vi "ClusterToDescriptiveStringGeneric.vi"(8 "error in":errorcluster, 11 "Cluster In":refnum<vi>) -> (0 "error out":errorcluster, 3 "String":string)   [LabVIEW 2023]
doc: "This VI turns a cluster (from reference) into a human/machine readable string."
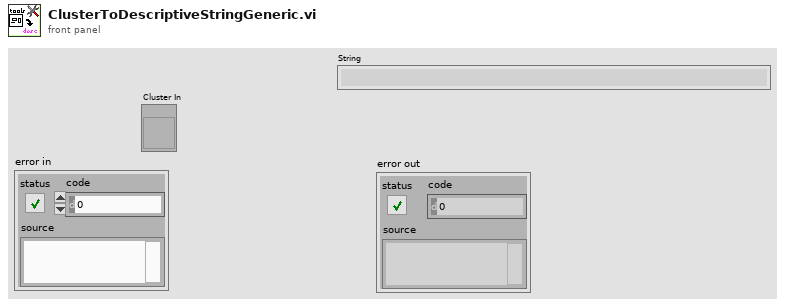
[diagram p1: front panel]
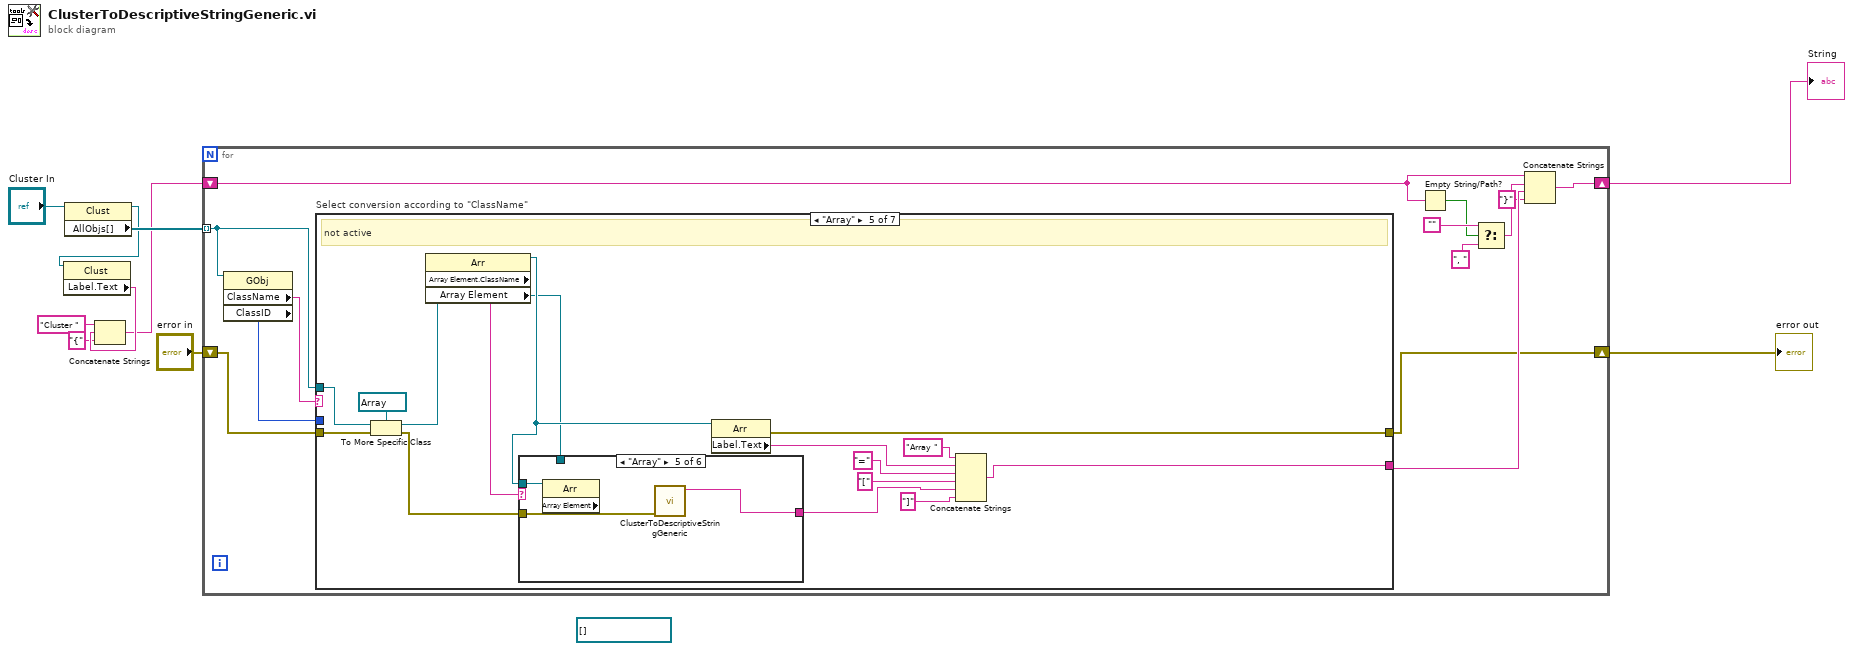
[diagram p0: block diagram]
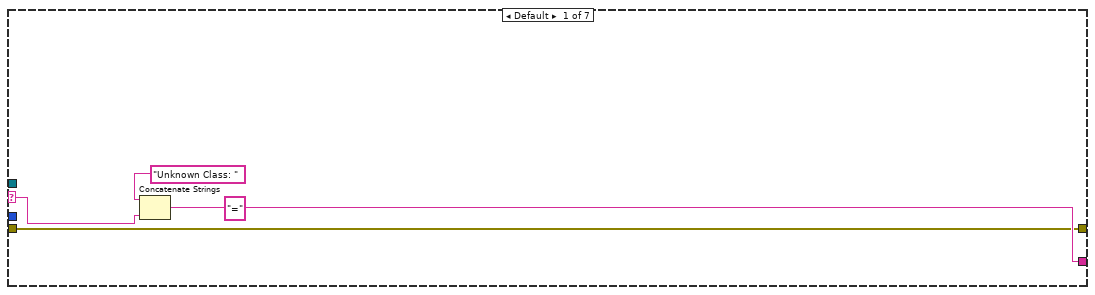
[diagram p2: hidden frame]
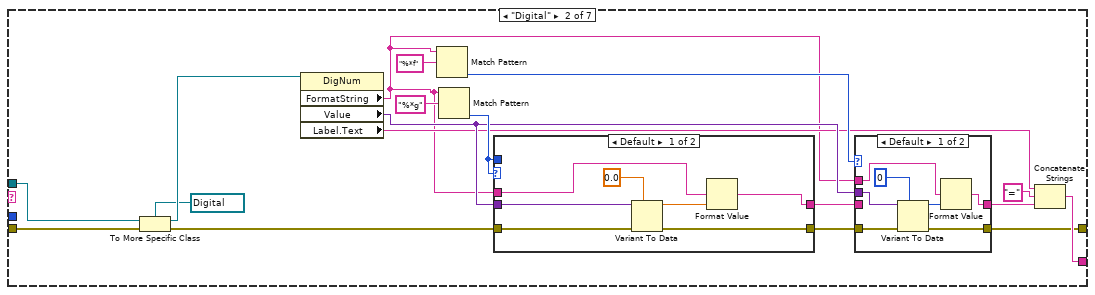
[diagram p3: hidden frame]
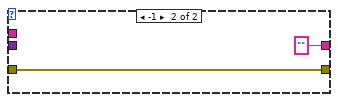
[diagram p5: hidden frame]
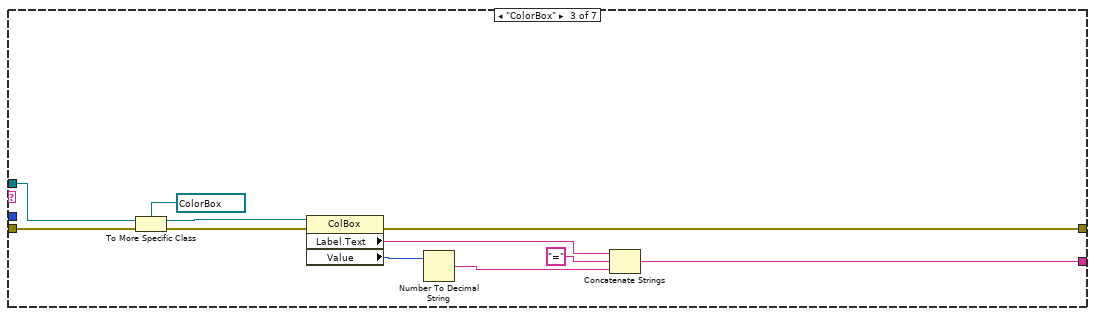
[diagram p6: hidden frame]
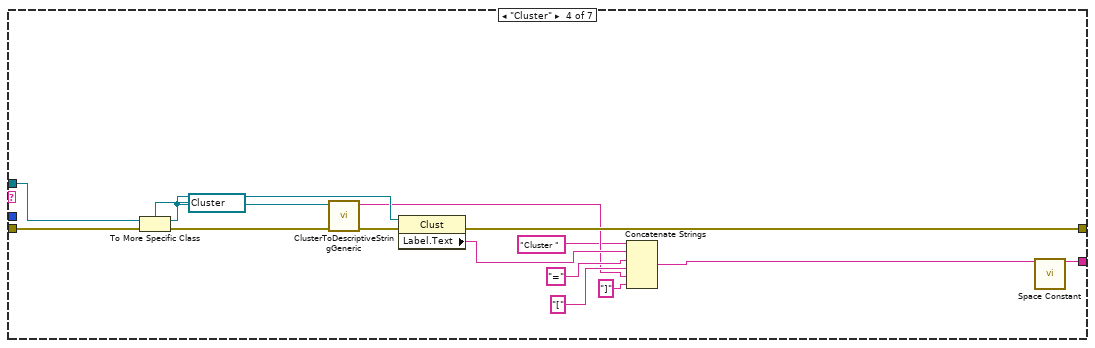
[diagram p7: hidden frame]
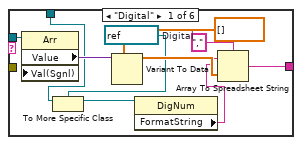
[diagram p8: hidden frame]
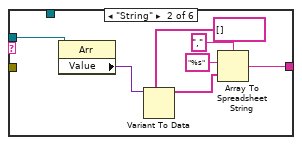
[diagram p9: hidden frame]
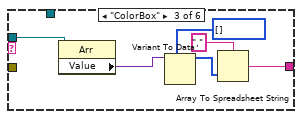
[diagram p10: hidden frame]
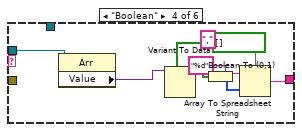
[diagram p11: hidden frame]
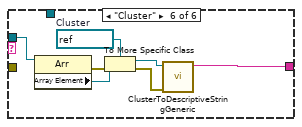
[diagram p12: hidden frame]
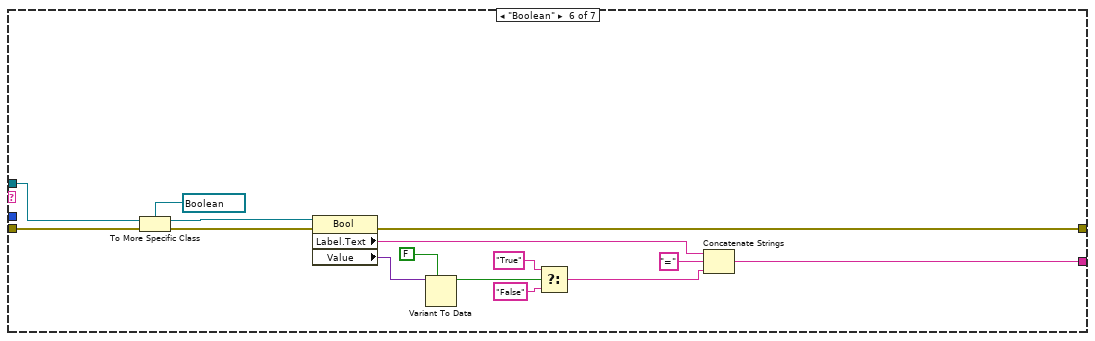
[diagram p13: hidden frame]
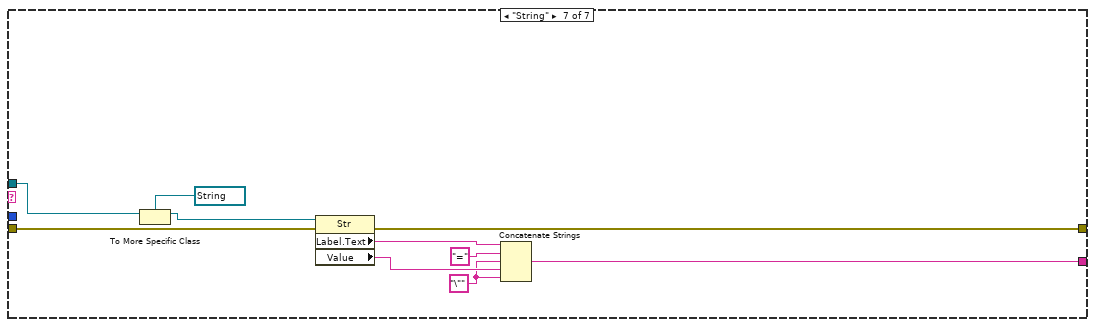
[diagram p14: hidden frame]
diagram:
  (unwired) refnum<vi>[] []
  n1 = property on="Property Node" class="Clust"(reference="Cluster In") -> (reference out=w5:refnum<vi>, "AllObjs[]"=w7:refnum<vi>[])  [unwired: 1 in, 1 out]
  n2 = property on="Property Node" class="Clust"(reference=w5) -> ("Label.Text"=w3:string)  [unwired: 1 in, 2 out]
  n3 = Concatenate Strings("Cluster " ("string"), w3, "{" ("string")) -> (w1:string)
  n4 = for {
    tunnel: w7 -> [w22] mode=indexing
    shift-right: [w23] -> w10
    shift-left: w1 -> [w13]
    shift-right: [w16] -> w8
    shift-left: "error in" -> [w15]
    n5 = property on="Property Node" class="GObj"(reference=w22) -> ("ClassName"=w20:string, "ClassID"=w21:u32)  [unwired: 1 in, 2 out]
    n6 = case "Select conversion according to \"ClassName\"" shown="\"Array\"" w20 {
      selector: w20 -> [w26 _ _ _ _ _ _]
      tunnel: [w25 w36 w71 w87 w103 w158 w169] -> w19
      tunnel: w22 -> [_ w46 w75 w89 w105 w161 w171]
      tunnel: w21 -> [_ _ _ _ _ _ _]
      tunnel: [w24 w30 w67 w84 w101 w149 w163] -> w16
      tunnel: w15 -> [w24 w33 w65 w83 w100 w147 w162]
      frame Default {
        n7 = Concatenate Strings("Unknown Class: ", "=", w26) -> (w25:string)
      }
      frame "Digital" {
        n8 = To More Specific Class(target class=refnum<vi> refnum ("567"), reference=w46, error in=w33) -> (specific class reference=w45:refnum<vi>, error out=w32:errorcluster)
        n9 = property on="Property Node" class="DigNum"(reference=w45) -> ("FormatString"=w35:string, "Value"=w42:variant, "Label.Text"=w38:string)  [unwired: 1 in, 2 out]
        n10 = Match Pattern(string=w35, regular expression="%*f") -> (offset past match=w39:i32)  [unwired: 1 in, 3 out]
        n11 = Match Pattern(string=w35, regular expression="%*g") -> (offset past match=w44:i32)  [unwired: 1 in, 3 out]
        n12 = case shown="Default" w44 {
          tunnel: w44 -> [_ _]
          tunnel: w42 -> [w62 _]
          tunnel: [w60 "" ("output string")] -> w43
          tunnel: w35 -> [w59 _]
          tunnel: w32 -> [w58 w63]
          tunnel: [w57 w63] -> w31
          frame Default {
            n13 = Variant To Data(error in=w58, type=0.0, Variant=w62) -> (data=w61:dbl, error out=w57:errorcluster)
            n14 = Format Value(format string=w59, value (0)=w61) -> (output string=w60:string)  [unwired: 1 in]
          }
          frame -1 {
          }
        }
        n15 = case shown="Default" w39 {
          tunnel: w42 -> [w53 _]
          tunnel: w43 -> [_ w55]
          tunnel: [w51 w55] -> w37
          tunnel: w35 -> [w50 _]
          tunnel: w31 -> [w49 w54]
          tunnel: [w48 w54] -> w30
          frame Default {
            n16 = Variant To Data(error in=w49, type=0, Variant=w53) -> (data=w52:i32, error out=w48:errorcluster)
            n17 = Format Value(format string=w50, value (0)=w52) -> (output string=w51:string)  [unwired: 1 in]
          }
          frame -1 {
          }
        }
        n18 = Concatenate Strings(w38, "=" ("string"), w37) -> (w36:string)
      }
      frame "ColorBox" {
        n19 = To More Specific Class(target class=refnum<vi> refnum ("Left"), reference=w75, error in=w65) -> (specific class reference=w74:refnum<vi>, error out=w66:errorcluster)
        n20 = property on="Property Node" class="ColBox"(reference=w74, error in=w66) -> (error out=w67:errorcluster, "Label.Text"=w72:string, "Value"=w69:u32)  [unwired: 1 out]
        n21 = Number To Decimal String(number=w69) -> (decimal integer string=w73:string)  [unwired: 1 in]
        n22 = Concatenate Strings(w72, "=" ("string"), w73) -> (w71:string)
      }
      frame "Cluster" {
        n23 = To More Specific Class(target class=refnum<vi> refnum ("Left"), reference=w89, error in=w83) -> (specific class reference=w81:refnum<vi>, error out=w82:errorcluster)
        n24 = call "ClusterToDescriptiveStringGeneric.vi"("error in"=w82, "Cluster In"=w81) -> ("error out"=w80:errorcluster, "String"=w78:string)  [unwired: 8 in]
        n25 = property on="Property Node" class="Clust"(reference=w81, error in=w80) -> (error out=w84:errorcluster, "Label.Text"=w88:string)  [unwired: 1 out]
        n26 = Concatenate Strings("Cluster " ("string"), w88, "=" ("string"), "[" ("string"), w78, "]" ("string")) -> (w87:string)
        n27 = call <vilib>:"Space Constant.vi"() -> ()  [unwired: 1 out]
      }
      frame "Array" {
        # "not active"
        n28 = To More Specific Class(target class=refnum<vi> refnum ("Left"), reference=w105, error in=w100) -> (specific class reference=w95:refnum<vi>, error out=w91:errorcluster)
        n29 = property on="Property Node" class="Arr"(reference=w95) -> (reference out=w93:refnum<vi>, "Array Element.ClassName"=w94:string, "Array Element"=w90:refnum<vi>)  [unwired: 1 in, 1 out]
        n30 = case shown="\"Array\"" w94 {
          tunnel: w93 -> [w115 w122 w128 w136 w137 w146]
          tunnel: [w111 w118 w124 w129 w138 w142] -> w92
          tunnel: w91 -> [_ _ _ _ w139 _]
          tunnel: w90 -> [w109 _ _ _ _ _]
          frame "Digital" {
            w108 = refnum<vi> refnum  # Digital
            n31 = property on="Property Node" class="Arr" props=["Value", "Val(Sgnl)"](reference=w115) -> ("Value"=w114:variant)  [unwired: 2 in, 2 out]
            n32 = To More Specific Class(target class=w108, reference=w109) -> (specific class reference=w107:refnum<vi>)  [unwired: 1 in, 1 out]
            n33 = Variant To Data(type=dbl[] [], Variant=w114) -> (data=w112:dbl[])  [unwired: 1 in, 1 out]
            n34 = property on="Property Node" class="DigNum"(reference=w107) -> ("FormatString"=w106:string)  [unwired: 1 in, 2 out]
            n35 = Array To Spreadsheet String(delimiter (Tab)=",", array=w112, 3:w106) -> (spreadsheet string=w111:string)
          }
          frame "String" {
            n36 = property on="Property Node" class="Arr"(reference=w122) -> ("Value"=w121:variant)  [unwired: 1 in, 2 out]
            n37 = Variant To Data(type=string[] [], Variant=w121) -> (data=w119:string[])  [unwired: 1 in, 1 out]
            n38 = Array To Spreadsheet String(delimiter (Tab)=",", array=w119, 3:"%s" ("format string")) -> (spreadsheet string=w118:string)
          }
          frame "ColorBox" {
            n39 = property on="Property Node" class="Arr"(reference=w128) -> ("Value"=w127:variant)  [unwired: 1 in, 2 out]
            n40 = Variant To Data(type=u32[] [], Variant=w127) -> (data=w125:u32[])  [unwired: 1 in, 1 out]
            n41 = Array To Spreadsheet String(delimiter (Tab)=",", array=w125) -> (spreadsheet string=w124:string)  [unwired: 1 in]
          }
          frame "Boolean" {
            n42 = property on="Property Node" class="Arr"(reference=w136) -> ("Value"=w135:variant)  [unwired: 1 in, 2 out]
            n43 = Variant To Data(type=bool[] [], Variant=w135) -> (data=w133:bool[])  [unwired: 1 in, 1 out]
            n44 = Boolean To (0,1)(Boolean=w133) -> (0, 1=w132:i16[])
            n45 = Array To Spreadsheet String(delimiter (Tab)=",", array=w132, 3:"%d" ("format string")) -> (spreadsheet string=w129:string)
          }
          frame "Array" {
            n46 = property class="Arr" props=["Array Element"](reference=w137) -> ()  [unwired: 1 in, 3 out]
            n47 = call "ClusterToDescriptiveStringGeneric.vi"("error in"=w139) -> ("String"=w138:string)  [unwired: 9 in, 1 out]
          }
          frame "Cluster" {
            w144 = refnum<vi> refnum  # Cluster
            n48 = property class="Arr"(reference=w146) -> (error out=w140:errorcluster, "Array Element"=w145:refnum<vi>)  [unwired: 1 in, 1 out]
            n49 = To More Specific Class(target class=w144, reference=w145, error in=w140) -> (specific class reference=w143:refnum<vi>, error out=w141:errorcluster)
            n50 = call "ClusterToDescriptiveStringGeneric.vi"("error in"=w141, "Cluster In"=w143) -> ("String"=w142:string)  [unwired: 8 in, 1 out]
          }
        }
        n51 = property on="Property Node" class="Arr"(reference=w93) -> (error out=w101:errorcluster, "Label.Text"=w104:string)  [unwired: 1 in, 1 out]
        n52 = Concatenate Strings("Array " ("string"), w104, "=" ("string"), "[" ("string"), w92, "]" ("string")) -> (w103:string)
      }
      frame "Boolean" {
        n53 = To More Specific Class(target class=refnum<vi> refnum ("Left"), reference=w161, error in=w147) -> (specific class reference=w160:refnum<vi>, error out=w148:errorcluster)
        n54 = property on="Property Node" class="Bool"(reference=w160, error in=w148) -> (error out=w149:errorcluster, "Label.Text"=w159:string, "Value"=w155:variant)  [unwired: 1 out]
        n55 = Variant To Data(type=FALSE ("x = y?"), Variant=w155) -> (data=w153:bool)  [unwired: 1 in, 1 out]
        n56 = Select(t="True" ("Label.Text"), s=w153, f="False" ("Label.Text")) -> (s? t:f=w150:string)
        n57 = Concatenate Strings(w159, "=" ("string"), w150) -> (w158:string)
      }
      frame "String" {
        w166 = "\"" ("string")
        n58 = To More Specific Class(target class=refnum<vi> refnum ("Numeric"), reference=w171) -> (specific class reference=w170:refnum<vi>)  [unwired: 1 in, 1 out]
        n59 = property on="Property Node" class="Str"(reference=w170, error in=w162) -> (error out=w163:errorcluster, "Label.Text"=w165:string, "Value"=w167:string)  [unwired: 1 out]
        n60 = Concatenate Strings(w165, "=" ("string"), w166, w167, w166) -> (w169:string)
      }
    }
    n61 = Empty String/Path?(string/path=w13) -> (empty?=w12:bool)
    n62 = Select(t="" ("Empty String Constant"), s=w12, f=", " ("string")) -> (s? t:f=w17:string)
    n63 = Concatenate Strings(w13, w17, w19, "}" ("string")) -> (w23:string)
  }
  "String" <- w10
  "error out" <- w8
